vi "Start AO.vi"(8 "error in (no error)":errorcluster, 10 "AO []":waveform(dbl)[](array[waveform]), 11 "DAQmx in":refnum<class "DAQmx.lvclass">) -> (0 "error out":errorcluster, 3 "DAQmx out":refnum<class "DAQmx.lvclass">)   [LabVIEW 2019, in "DAQmx.lvclass"]
uses:
  DAQmx.lvclass
  DAQmx.lvclass/DAQmx.ctl
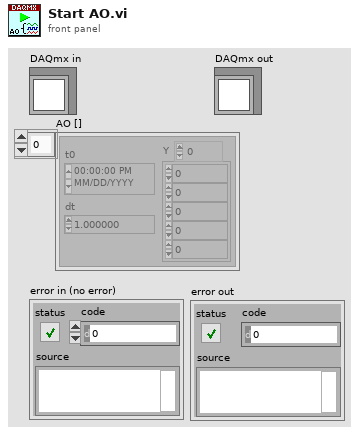
[diagram p1: front panel]
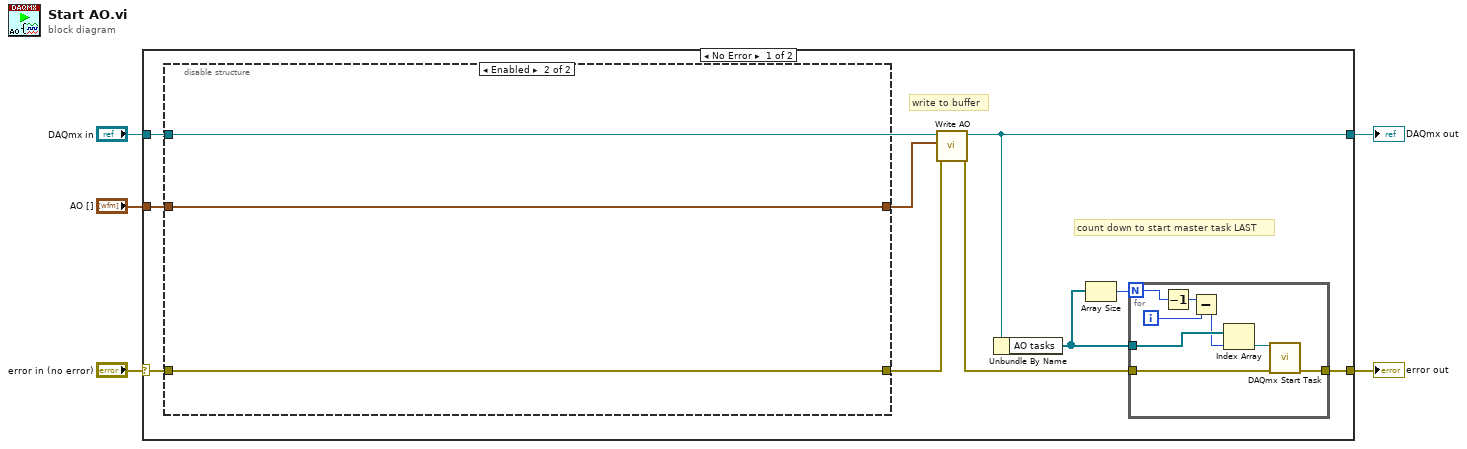
[diagram p0: block diagram]
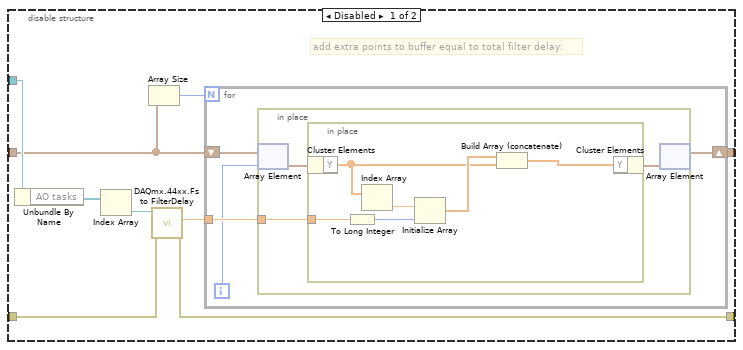
[diagram p2: hidden frame]
diagram:
  n1 = case shown="No Error" "error in (no error)" {
    selector: "error in (no error)" -> [w7 w49]
    tunnel: [w15 w49] -> w5
    tunnel: "DAQmx in" -> [w13 w48]
    tunnel: [w11 w48] -> w2
    tunnel: "AO []" -> [w10 _]
    frame No Error {
      # "write to buffer"
      # "count down to start master task LAST"
      n2 = disable-structure shown="Enabled" {
        disable-tunnel: w13 -> [w24 _]
        disable-tunnel: w10 -> [w23 w39]
        disable-tunnel: [w18 w39] -> w8
        disable-tunnel: w7 -> [w17 w38]
        disable-tunnel: [w16 w38] -> w6
        frame Disabled {
          # "add extra points to buffer equal to total filter delay:"
          n3 = Unbundle By Name(w24) -> ("AO tasks"=w21:refnum<k21>[])
          n4 = Index Array(array=w21) -> (element=w20:refnum<k21>)  [unwired: 1 in]
          n5 = Array Size(array=w23) -> (size(s)=w22:i32)
          n6 = call "DAQmx.44xx.Fs to FilterDelay.vi"("error in (no error)"=w17, "Refnum in"=w20) -> ("error out"=w16:errorcluster, "Filter Delay (samples)"=w19:dbl)  [unwired: 7 in, 1 out]
          n7 = for {
            N: w22 -> [_]
            shift-right: [w27] -> w18
            shift-left: w23 -> [w28]
            tunnel: w19 -> [w26]
            i -> [w25]
            n8 = in-place {
              in-place-border: w26 -> [w30]
              n9 = in-place-array #1(w28, w25) -> (w31:waveform(dbl))
              n10 = in-place {
                in-place-border: w30 -> [w36]
                n11 = in-place-cluster #2(w31) -> ("Y"=w34:dbl[])
                n12 = To Long Integer(number=w36) -> (32bit integer=w32:i32)
                n13 = Index Array(array=w34) -> (element=w37:dbl)  [unwired: 1 in]
                n14 = Initialize Array(w37, w32) -> (w35:dbl[])
                n15 = Build Array (concatenate)(w35, w34) -> (w33:dbl[])
                n16 = in-place-cluster #2("Y"=w33) -> (w29:waveform(dbl))
              }
              n17 = in-place-array #1(w29) -> (w27:waveform(dbl)[])  [unwired: 1 out]
            }
          }
        }
        frame Enabled {
        }
      }
      n18 = call "Write AO.vi"("error in (no error)"=w6, "AO []"=w8, "DAQmx in"=w13) -> ("error out"=w12:errorcluster, "DAQmx out"=w11:refnum<class "DAQmx.lvclass">)  [unwired: 5 in, 2 out]
      n19 = Unbundle By Name(w11) -> ("AO tasks"=w9:refnum<k21>[])
      n20 = Array Size(array=w9) -> (size(s)=w14:i32)
      n21 = for {
        N: w14 -> [w45]
        tunnel: w9 -> [w46]
        tunnel: [w47] -> w15
        tunnel: w12 -> [w41]
        i -> [w42]
        n22 = Decrement(x=w45) -> (x-1=w44:i32)
        n23 = Subtract(x=w44, y=w42) -> (x-y=w43:i32)
        n24 = Index Array(array=w46, index=w43) -> (element=w40:refnum<k21>)
        n25 = call <vilib>:"DAQmx Start Task.vi"("task/channels in"=w40, "error in"=w41) -> ("error out"=w47:errorcluster)  [unwired: 12 in, 1 out]
      }
    }
    frame Error {
    }
  }
  "DAQmx out" <- w2
  "error out" <- w5
